vi "Create.vi"(7 "Direction":T1, 8 "error in (no error)":errorcluster, 9 "Custom Config Data":u8[](array[numeric]), 10 "Name":string, 11 "CIFFIFO in":refnum<class "CIF_CIPC_Fifo_DAQ.lvclass">) -> (0 "error out":errorcluster, 3 "CIFFIFO out":refnum<class "CIF_CIPC_Fifo_DAQ.lvclass">)   [LabVIEW 2021, in "CIF_CIPC_Fifo_DAQ.lvclass"]
uses:
  CIF_CIPC_Fifo_DAQ.lvclass
  CIF_CIPC_Fifo_DAQ.lvclass/CIF_CIPC_Fifo_DAQ.ctl
  CIFChannels/CIFChannels.lvclass
  CIFChannels/Typedef/Disconnect Behavior.ctl
  CIFChannels/Typedef/Channel State.ctl
  <vilib>/CIF Foundation/CIF Utilities/Statistics/I64/Stats_I64_CIF_U.lvclass
  ChannelCommon/ChannelCommon.lvlib
  ChannelCommon/typedef/Channel Pattern.ctl
  35849dc3-58aa-4d75-b906-fe3df34869a7.vi
  <vilib>/CIF Foundation/CIF CIPC/TypeDefs/Backpressure References.ctl
  <vilib>/CIF Foundation/CIF CIPC/CIF_NI_CIPC.lvlib
  CIF_CIPC_Chan/Typedef/Buffer Configuration Data.ctl
  CIF_CIPC_Chan/CIF_CIPC_Chn.lvclass
  9be4d617-3037-4515-bcea-2a1e3727d04e.vi
  D:/dev/Packages/CIF_Channels_Core/src/CIPC_Channels/CIF_CIPC_Chan/CIF_CIPC_Chn.lvclass
  D:/dev/Packages/CIF_Channels_Core/src/CIFChannels/CIFChannels.lvclass
  D:/dev/Packages/CIF_Channels_Core/src/CIPC_Channels/FIFO_DAQ/CIF_CIPC_Fifo_DAQ.lvclass
  CIFChannels/Typedef/Direction.ctl
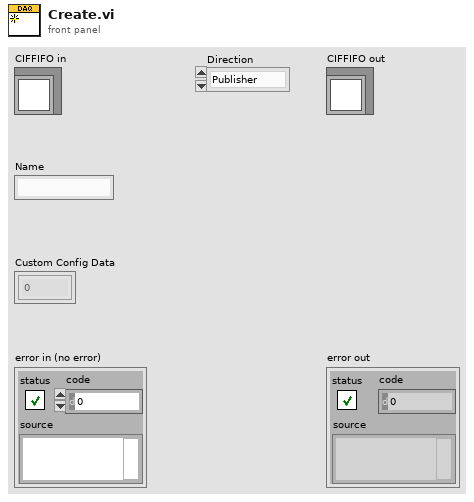
[diagram p1: front panel]
types:
  T1 = typedef "CIFChannels.lvclass/Direction.ctl" = enum16{"Publisher", "Subscriber"}
  T2 = typedef "CIFChannels.lvclass/Disconnect Behavior.ctl" = enum16{"Default value", "Last value", "Error with default"}
  T3 = typedef "CIFChannels.lvclass/Channel State.ctl" = enum16{"Creating", "Disconnected", "Connecting", "Connected", "Destroyed"}
  T4 = typedef "ChannelCommon.lvlib/Channel Pattern.ctl" = enum16{"Unknown", "Tag", "FIFO", "MultiFIFO", "BackpressureFIFO"}
  T5 = typedef "CIF_CIPC_Chn.lvclass/Buffer Configuration Data.ctl" = cluster{"Total Size":u32, "Read Size":u32, "Read Offset":u32, "CIPC BP References":T6, "Override CIPC Name":string, "Encoder Data":string}
  T6 = typedef "CIF_NI_CIPC.lvlib/Backpressure References.ctl" = cluster{"CIPC Reference":u64, "CIPC BP Reference":u64}
  T7 = typedef "CIF_NI_CIPC.lvlib/Encoder Info.ctl" = cluster{"Name":string, "Version":i32, "Data":string}
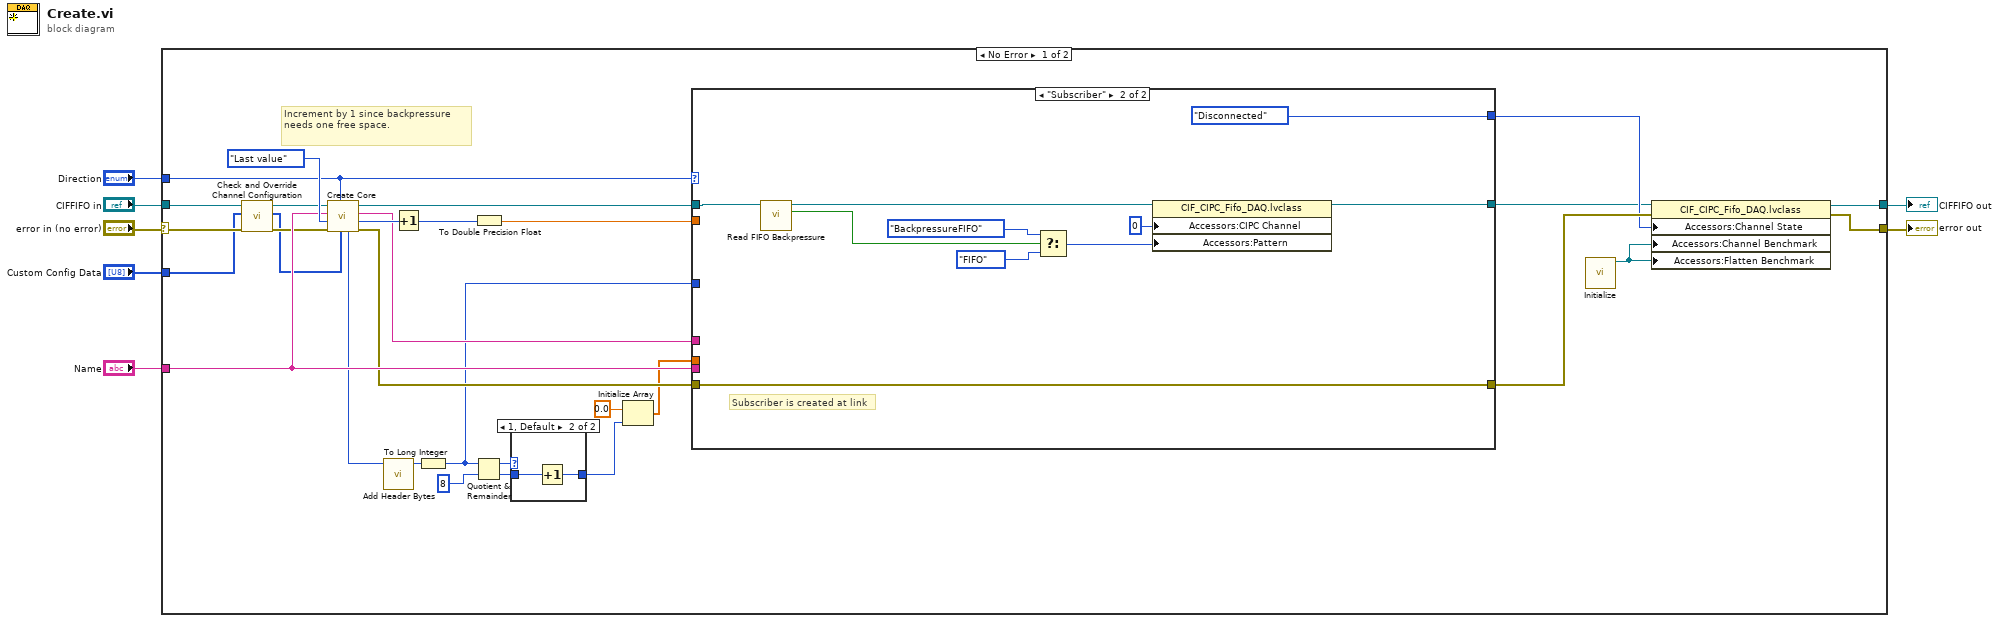
[diagram p0: block diagram]
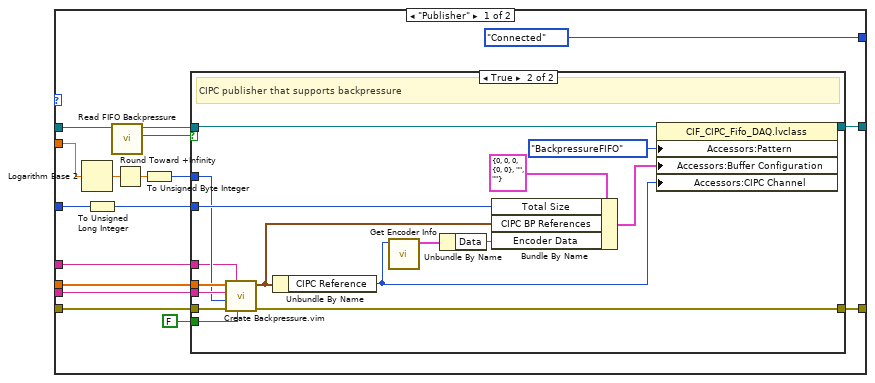
[diagram p3: hidden frame]
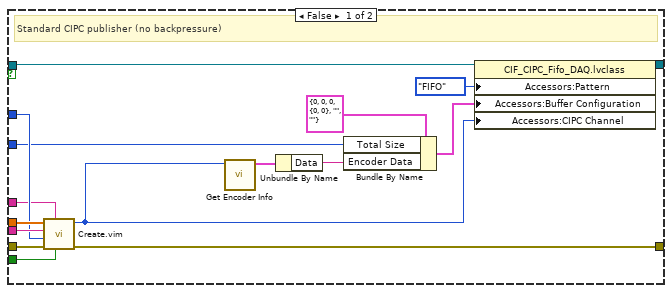
[diagram p4: hidden frame]
diagram:
  n1 = case shown="No Error" "error in (no error)" {
    selector: "error in (no error)" -> [w26 w102]
    tunnel: [w36 w102] -> w6
    tunnel: [w32 w101] -> w1
    tunnel: "CIFFIFO in" -> [w27 w101]
    tunnel: "Name" -> [w35 _]
    tunnel: "Direction" -> [w31 _]
    tunnel: "Custom Config Data" -> [w23 _]
    frame No Error {
      # "Increment by 1 since backpressure needs one free space."
      n2 = call-dynamic "Check and Override Channel Configuration.vi"("error in (no error)"=w26, "Custom Config Data in"=w23, "CIFFIFO in"=w27) -> ("error out"=w24:errorcluster, "Custom Config Data out"=w22:u8[], "CIFFIFO out"=w25:refnum<class "CIF_CIPC_Fifo_DAQ.lvclass">)  [unwired: 6 in]
      n3 = call "Create Core.vi"("Custom Config Data"=w22, "Direction"=w31, "error in (no error)"=w24, "Disconnect Behavior"=Disconnect_Behavior."Last value", "Name"=w35, "CIFChannels in"=w25) -> ("error out"=w34:errorcluster, "Messages"=w17:u64, "Channel Type"=w15:string, "CIFChannels out"=w19:refnum<class "CIF_CIPC_Fifo_DAQ.lvclass">, "Bytes/Msg"=w14:u64)  [unwired: 1 in]
      n4 = call "Add Header Bytes.vi"("Bytes/Msg"=w14) -> ("Bytes/Msg with header"=w18:u64)  [unwired: 3 in]
      n5 = Increment(x=w17) -> (x+1=w16:u64)
      n6 = To Long Integer(number=w18) -> (32bit integer=w13:i32)
      n7 = Quotient & Remainder(x=w13, y=8) -> (x-y*floor(x/y)=w11:i32, floor(x/y)=w10:i32)
      n8 = To Double Precision Float(number=w16) -> (double precision float=w20:dbl)
      n9 = case shown="1, Default" w11 {
        tunnel: w10 -> [w38 w40]
        tunnel: [w38 w39] -> w9
        frame 0 {
        }
        frame 1, Default {
          n10 = Increment(x=w40) -> (x+1=w39:i32)
        }
      }
      n11 = Initialize Array(0.0 ("Numeric"), w9) -> (w21:dbl[])
      n12 = case shown="\"Subscriber\"" w31 {
        tunnel: w35 -> [w53 _]
        tunnel: w34 -> [w55 w99]
        tunnel: [w56 w99] -> w33
        tunnel: [Channel_State."Connected" ("Channel State") Channel_State."Disconnected" ("Channel State")] -> w30
        tunnel: w20 -> [w50 _]
        tunnel: w21 -> [w52 _]
        tunnel: w19 -> [w47 w93]
        tunnel: w13 -> [w44 _]
        tunnel: [w42 w98] -> w8
        tunnel: w15 -> [w41 _]
        frame "Publisher" {
          n13 = Logarithm Base 2(1:w50) -> (0:w51:dbl)
          n14 = To Unsigned Long Integer(number=w44) -> (unsigned 32bit integer=w43:u32)
          n15 = call "Read FIFO Backpressure.vi"("CIFChannels in"=w47) -> ("Backpressure"=w45:bool, "CIFChannels out"=w46:refnum<class "CIF_CIPC_Fifo_DAQ.lvclass">)  [unwired: 8 in, 1 out]
          n16 = Round Toward +Infinity(x=w51) -> (ceil(x): smallest int >= x=w49:dbl)
          n17 = To Unsigned Byte Integer(number=w49) -> (unsigned 8bit integer=w48:u8)
          n18 = case shown="True" w45 {
            tunnel: [w73 w79] -> w56
            tunnel: w55 -> [w72 w80]
            tunnel: FALSE ("Prepend Array Size") -> [w71 w83]
            tunnel: w53 -> [w70 w82]
            tunnel: w52 -> [w69 w84]
            tunnel: w48 -> [w68 w81]
            tunnel: w46 -> [w67 w90]
            tunnel: w43 -> [w65 w88]
            tunnel: [w61 w85] -> w42
            tunnel: w41 -> [w60 w76]
            frame False {
              # "Standard CIPC publisher (no backpressure)"
              n19 = call "Create.vim"("Prepend Array Size"=w71, "Description"=w60, "error in (no error)"=w72, "Buffer Size N (2^N)"=w68, "Name in"=w70, "Data Type"=w69) -> ("error out"=w73:errorcluster, "CIPC Reference"=w62:u64)  [unwired: 2 in, 2 out]
              n20 = call <vilib>:"Get Encoder Info.vi"("CIPC Reference"=w62) -> ("Encoder Info"=w64:T7)  [unwired: 9 in, 1 out]
              n21 = Unbundle By Name(w64) -> ("Data"=w63:string)
              n22 = Bundle By Name(cluster=T5 {"Total Size"=0, "Read Size"=0, "Read Offset"=0, "CIPC BP References"={"CIPC Reference"=0, "CIPC BP Reference"=0}, "Override CIPC Name"="", "Encoder Data"=""} ("Buffer Configuration"), "Total Size"=w65, "Encoder Data"=w63) -> (w59:T5)
              n23 = property class="CIF_CIPC_Fifo_DAQ.lvclass"(reference=w67, "Accessors:Pattern"=Channel_Pattern."FIFO" ("Pattern"), "Accessors:Buffer Configuration"=w59, "Accessors:CIPC Channel"=w62) -> (reference out=w61:refnum<class "CIF_CIPC_Fifo_DAQ.lvclass">)  [unwired: 1 in, 1 out]
            }
            frame True {
              # "CIPC publisher that supports backpressure"
              n24 = call "Create Backpressure.vim"("Prepend Array Size"=w83, "Description"=w76, "error in (no error)"=w80, "Buffer Size N (2^N)"=w81, "Name in"=w82, "Data Type"=w84) -> ("error out"=w79:errorcluster, "CIPC BP References"=w77:T6)  [unwired: 2 in, 2 out]
              n25 = Unbundle By Name(w77) -> ("CIPC Reference"=w78:u64)
              n26 = call <vilib>:"Get Encoder Info.vi"("CIPC Reference"=w78) -> ("Encoder Info"=w87:T7)  [unwired: 9 in, 1 out]
              n27 = Unbundle By Name(w87) -> ("Data"=w86:string)
              n28 = Bundle By Name(cluster=T5 {"Total Size"=0, "Read Size"=0, "Read Offset"=0, "CIPC BP References"={"CIPC Reference"=0, "CIPC BP Reference"=0}, "Override CIPC Name"="", "Encoder Data"=""} ("Buffer Configuration"), "Total Size"=w88, "CIPC BP References"=w77, "Encoder Data"=w86) -> (w75:T5)
              n29 = property class="CIF_CIPC_Fifo_DAQ.lvclass"(reference=w90, "Accessors:Pattern"=Channel_Pattern."BackpressureFIFO" ("Pattern"), "Accessors:Buffer Configuration"=w75, "Accessors:CIPC Channel"=w78) -> (reference out=w85:refnum<class "CIF_CIPC_Fifo_DAQ.lvclass">)  [unwired: 1 in, 1 out]
            }
          }
        }
        frame "Subscriber" {
          # "Subscriber is created at link"
          n30 = call "Read FIFO Backpressure.vi"("CIFChannels in"=w93) -> ("Backpressure"=w94:bool, "CIFChannels out"=w92:refnum<class "CIF_CIPC_Fifo_DAQ.lvclass">)  [unwired: 8 in, 1 out]
          n31 = Select(t=Channel_Pattern."BackpressureFIFO" ("Pattern"), s=w94, f=Channel_Pattern."FIFO" ("Pattern")) -> (s? t:f=w91:T4)
          n32 = property class="CIF_CIPC_Fifo_DAQ.lvclass"(reference=w92, "Accessors:CIPC Channel"=u64 0 ("CIPC Channel"), "Accessors:Pattern"=w91) -> (reference out=w98:refnum<class "CIF_CIPC_Fifo_DAQ.lvclass">)  [unwired: 1 in, 1 out]
        }
      }
      n33 = call <vilib>:"Initialize.vi"() -> ("Stats_I64_CIF_U out"=w28:refnum<class "Stats_I64_CIF_U.lvclass">)  [unwired: 10 in, 1 out]
      n34 = property class="CIF_CIPC_Fifo_DAQ.lvclass"(reference=w8, error in=w33, "Accessors:Channel State"=w30, "Accessors:Channel Benchmark"=w28, "Accessors:Flatten Benchmark"=w28) -> (reference out=w32:refnum<class "CIF_CIPC_Fifo_DAQ.lvclass">, error out=w36:errorcluster)
    }
    frame Error {
    }
  }
  "error out" <- w6
  "CIFFIFO out" <- w1
